vi "string_to_common_trigger.vi"(8 "error in (no error)":errorcluster, 10 "trigger string":string, 11 "GenericToplevelComponent in":refnum<class "GenericToplevelComponent.lvclass">) -> (0 "error out":errorcluster, 2 "trigger":T1, 3 "GenericToplevelComponent out":refnum<class "GenericToplevelComponent.lvclass">)   [LabVIEW 2010, in "GenericToplevelComponent.lvclass"]
uses:
  GenericToplevelComponent.lvclass
  common_trigger_enum.ctl
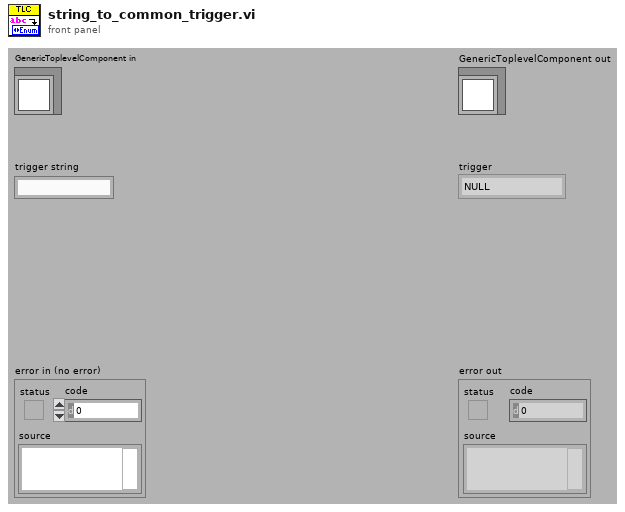
[diagram p1: front panel]
types:
  T1 = typedef "GenericToplevelComponent.lvclass/common_trigger_enum.ctl" = enum16{"NULL", "initialise", "terminate", "fetch command", "fetch data", "attach observer", "register as observer", "detach observer", "acknowledge", "start", "stop", "sweep started", "sweep finished", "experiment started", "experiment stopped"}
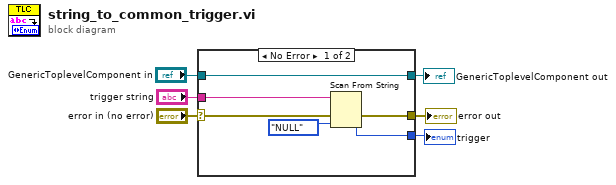
[diagram p0: block diagram]
diagram:
  n1 = case shown="No Error" "error in (no error)" {
    selector: "error in (no error)" -> [w11 w14]
    tunnel: [w10 w14] -> w5
    tunnel: [w12 w13] -> w3
    tunnel: "GenericToplevelComponent in" -> [w12 w13]
    tunnel: "trigger string" -> [w9 _]
    tunnel: [w7 _] -> w1
    frame No Error {
      n2 = Scan From String(input string=w9, error in=w11, default 1=common_trigger_enum."NULL" ("trigger")) -> (error out=w10:errorcluster, output 1=w7:T1)  [unwired: 2 in, 2 out]
    }
    frame Error {
    }
  }
  "error out" <- w5
  "GenericToplevelComponent out" <- w3
  "trigger" <- w1
